vi "Get Palette Color Array.vi"(8 "error in (no error)":errorcluster, 11 "Image Display Palette Information":T1 {"Palette Type" items=["Grayscale", "Binary", "Gradient", "Rainbow", "Temperature", "User Defined", "Binary 16 Bit", "Gradient 16 Bit", "Rainbow 16 Bit", "Temperature 16 Bit", "User Defined 16 Bit"]}) -> (0 "error out":errorcluster, 3 "1D Color value array":T3(array[cluster]))   [LabVIEW 2021, in "Palette.lvlib"]
uses:
  Image Palette Information.ctl
  Image/Image Display Palette Type.ctl
  Palette.lvlib
  <vilib>/vision/NI_Vision_Development_Module.lvlib
  Image/Image.lvlib
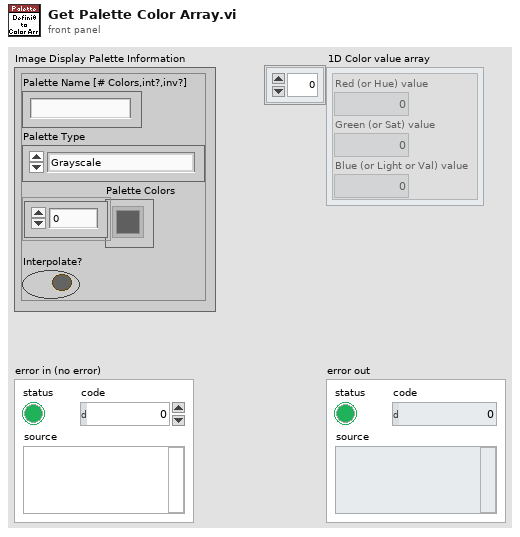
[diagram p1: front panel]
types:
  T1 = typedef "Palette.lvlib/Image Palette Information.ctl" = cluster{"Palette Name [# Colors,int?,inv?]":string, "Palette Type":T2, "Palette Colors":u32[], "Interpolate?":bool}
  T2 = typedef "Image.lvlib/Image Display Palette Type.ctl" = u32
  T3 = cluster{"Red (or Hue) value":u8, "Green (or Sat) value":u8, "Blue (or Light or Val) value":u8}[]
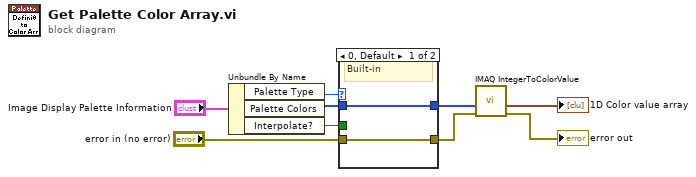
[diagram p0: block diagram]
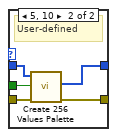
[diagram p2: hidden frame]
diagram:
  n1 = Unbundle By Name("Image Display Palette Information") -> ("Palette Type"=w6:T2, "Palette Colors"=w3:u32[], "Interpolate?"=w5:bool)
  n2 = case shown="0, Default" w6 {
    tunnel: w3 -> [w11 w16]
    tunnel: "error in (no error)" -> [w10 w15]
    tunnel: [w10 w14] -> w8
    tunnel: w5 -> [_ w13]
    tunnel: [w11 w12] -> w7
    frame 0, Default {
      # "Built-in"
    }
    frame 5, 10 {
      # "User-defined"
      n3 = call "Create 256 Values Palette.vi"("Error In"=w15, "Interpolate?"=w13, "Palette Colors in"=w16) -> ("Error Out"=w14:errorcluster, "1D U32 array"=w12:u32[])  [unwired: 5 in, 2 out]
    }
  }
  n4 = call "IMAQ IntegerToColorValue"("error in (no error)"=w8, "1D U32 array"=w7) -> ("1D Color value array"=→"1D Color value array":T3, "error out"=→"error out":errorcluster)  [unwired: 3 in, 2 out]
